vi "test_ShowAndHideUI.vi"(8 "error in (no error)":errorcluster, 11 "TestCase in":refnum<class "SMO.UI_TestCase.lvclass">) -> (0 "error out":errorcluster, 3 "TestCase out":refnum<class "SMO.UI_TestCase.lvclass">)   [LabVIEW 2013, in "SMO.UI_TestCase.lvclass"]
uses:
  SMO.UI_TestCase.lvclass
  SMO.UI_TestCase.lvclass/SMO.UI_TestCase.ctl
  <vilib>/addons/_JKI Toolkits/VI Tester/TestCase.llb/TestCase.lvclass
  src/SMO.UI/SMO.UI.lvclass
  src/SMO/SMO.lvclass
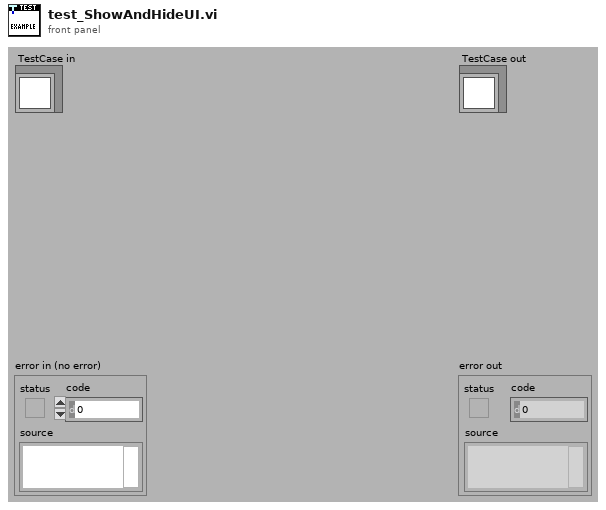
[diagram p1: front panel]
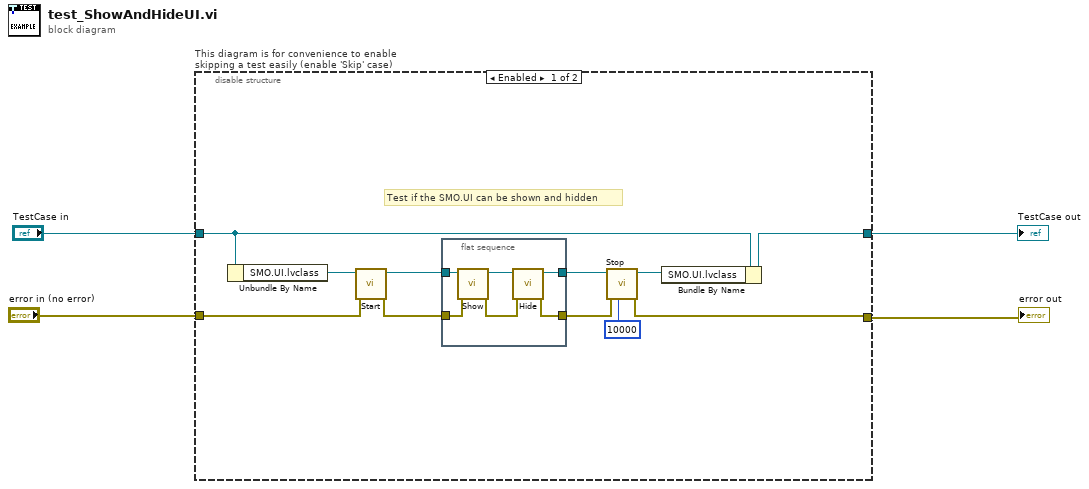
[diagram p0: block diagram]
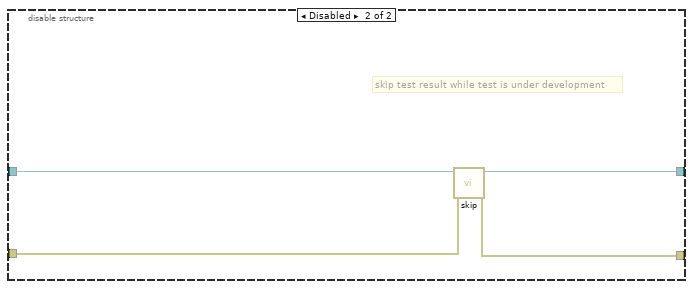
[diagram p2: hidden frame]
diagram:
  n1 = disable-structure "This diagram is for convenience to enable skipping a test easily (enable 'Skip' case)" shown="Enabled" {
    disable-tunnel: "TestCase in" -> [w15 w25]
    disable-tunnel: [w14 w23] -> w1
    disable-tunnel: [w5 w24] -> w3
    disable-tunnel: "error in (no error)" -> [w11 w22]
    frame Enabled {
      # "Test if the SMO.UI can be shown and hidden"
      n2 = Unbundle By Name(w15) -> ("SMO.UI.lvclass"=w13:refnum<class "SMO.UI.lvclass">)
      n3 = call "Start.vi"("error in (no error)"=w11, "SMO"=w13) -> ("error out"=w10:errorcluster, "SMO out"=w12:refnum<class "SMO.UI.lvclass">)  [unwired: 8 in]
      n4 = flat-sequence {
        tunnel: w12 -> [w21]
        tunnel: w10 -> [w20]
        tunnel: [w17] -> w8
        tunnel: [w16] -> w6
        frame #0 {
          n5 = call "Show.vi"("error in (no error)"=w20, "SMO.UI"=w21) -> ("error out"=w18:errorcluster, "SMO.UI out"=w19:refnum<class "SMO.UI.lvclass">)  [unwired: 8 in]
          n6 = call "Hide.vi"("error in (no error)"=w18, "SMO.UI"=w19) -> ("error out"=w16:errorcluster, "SMO.UI out"=w17:refnum<class "SMO.UI.lvclass">)  [unwired: 8 in]
        }
      }
      n7 = call "Stop.vi"("timeout in ms (-1)"=10000, "error in (no error)"=w6, "SMO"=w8) -> ("error out"=w5:errorcluster, "SMO out"=w7:refnum<class "SMO.UI.lvclass">)  [unwired: 7 in]
      n8 = Bundle By Name(cluster=w15, "SMO.UI.lvclass"=w7) -> (w14:refnum<class "SMO.UI_TestCase.lvclass">)
    }
    frame Disabled {
      # "skip test result while test is under development"
      n9 = call <vilib>:"skip.vi"("error in (no error)"=w22, "TestCase in"=w25) -> ("error out"=w24:errorcluster, "TestCase out"=w23:refnum<class "SMO.UI_TestCase.lvclass">)  [unwired: 8 in]
    }
  }
  "error out" <- w3
  "TestCase out" <- w1
